vi "Prober_MoveToLoad.vi"(8 "error in (no error)":errorcluster, 11 "AlessiRel6100 in":refnum<class "AlessiRel6100.lvclass">) -> (0 "error out":errorcluster, 3 "AlessiRel6100 out":refnum<class "AlessiRel6100.lvclass">)   [LabVIEW 2018, in "AlessiRel6100.lvclass"]
uses:
  AlessiRel6100.lvclass
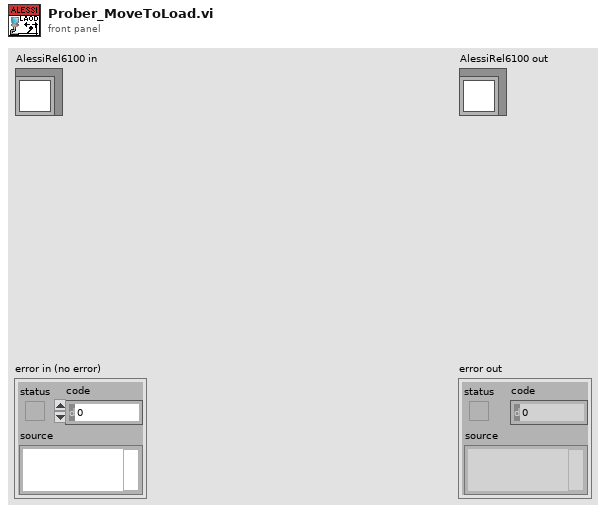
[diagram p1: front panel]
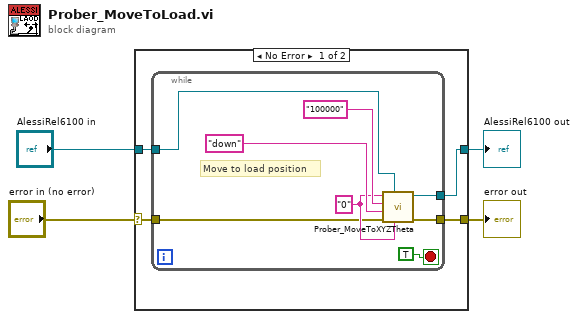
[diagram p0: block diagram]
diagram:
  n1 = case shown="No Error" "error in (no error)" {
    selector: "error in (no error)" -> [w8 w18]
    tunnel: [w7 w18] -> w1
    tunnel: "AlessiRel6100 in" -> [w5 w17]
    tunnel: [w6 w17] -> w3
    frame No Error {
      n2 = while {
        tunnel: w8 -> [w10]
        tunnel: [w12] -> w7
        tunnel: [w11] -> w6
        tunnel: w5 -> [w9]
        stop <- TRUE stop-if-true
        w13 = "0"
        # "Move to load position"
        n3 = call-dynamic "Prober_MoveToXYZTheta.vi"("Theta location [mdeg]"=w13, "AlessiRel6100 in"=w9, "error in (no error)"=w10, "Z location [µm]"="down", "Y location [µm]"="100000", "X location [µm]"=w13) -> ("error out"=w12:errorcluster, "AlessiRel6100 out"=w11:refnum<class "AlessiRel6100.lvclass">)  [unwired: 3 in, 1 out]
      }
    }
    frame Error {
    }
  }
  "error out" <- w1
  "AlessiRel6100 out" <- w3
